vi "ActDriveStraight.vi"(9 "FirstTime":bool, 10 "MaxSpeed (ft/s)":dbl, 11 "Dist (ft)":dbl) -> (1 "XSpeedDemand":dbl, 3 "Done":bool)   [LabVIEW 2020]
doc: "Robot will drive forward straight a set distance utilizing position control \n\nInputs:\n-- MaxSpeed -- Double -- in ft/s, the MaxSpeed the robot can go -- \n-- Dist (ft) -- Double -- Distance in feet you want the robot to go -- \n-- FirstTime -- Boolean -- Input true the first time this function is called, sets the target position -- \n\nOutputs:\n-- Done -- Bool -- has the robot reached its target distance\n-- LeftSpeedDemand -- Double -- Speed Demand for left drive train inorder to reach target -- \n-- RightSpeedDemand -- Double -- Speed Demand for left drive train inorder to reach target --"
uses:
  <vilib>/Rock Robotics/WPI/ThirdParty/JAS_Junk/TrajLib/Trajectory_Library.lvlib
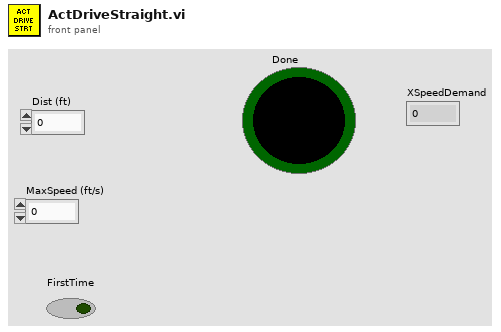
[diagram p1: front panel]
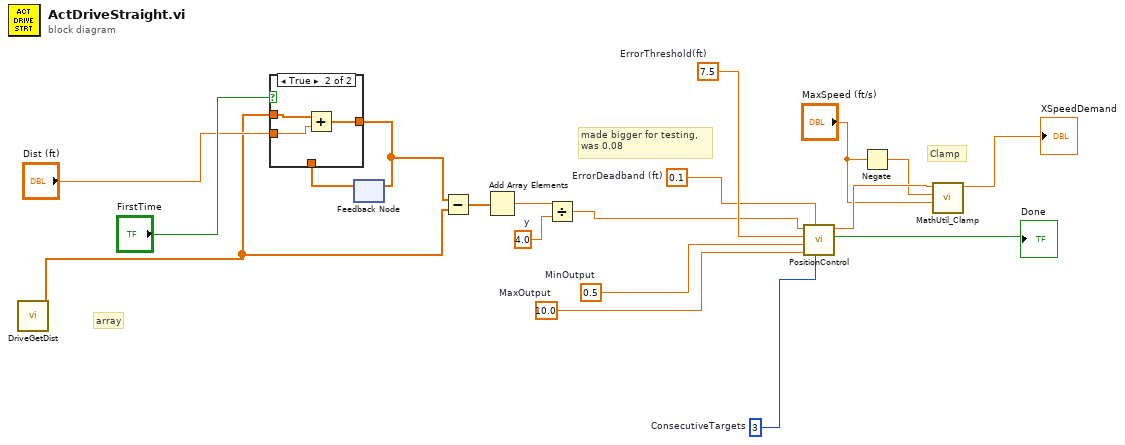
[diagram p0: block diagram]
diagram:
  w2 = 4.0  # y
  w10 = 10.0  # MaxOutput
  w11 = 0.5  # MinOutput
  w15 = 3  # ConsecutiveTargets
  w16 = 0.1  # ErrorDeadband (ft)
  w17 = 7.5  # ErrorThreshold(ft)
  # "made bigger for testing, \nwas 0.08"
  # "array"
  # "Clamp"
  n1 = call "DriveGetDist.vi"() -> ("ModuleTravelPosition"=w5:dbl[])  [unwired: 11 in]
  n2 = feedback #1() -> (w7:dbl[])  [unwired: 1 in]
  n3 = case shown="True" "FirstTime" {
    tunnel: "Dist (ft)" -> [_ w22]
    tunnel: w5 -> [_ w23]
    tunnel: [w20 w21] -> w6
    tunnel: w7 -> [w20 _]
    frame False {
    }
    frame True {
      n4 = Add(x=w23, y=w22) -> (x+y=w21:dbl[])
    }
  }
  n5 = feedback-in #1(w6) -> ()
  n6 = Subtract(x=w6, y=w5) -> (x-y=w4:dbl[])
  n7 = Add Array Elements(numeric array=w4) -> (sum=w3:dbl)
  n8 = Divide(x=w3, y=w2) -> (x/y=w1:dbl)
  n9 = call "PositionControl.vi"("ConsecutiveTargets"=w15, "ErrorDeadband"=w16, "MaxOutput"=w10, "MinOutput"=w11, "ErrorThreshold"=w17, "Error"=w1) -> ("OnTarget"=→"Done":bool, "OutputValue"=w14:dbl)  [unwired: 3 in, 1 out]
  n10 = Negate(x="MaxSpeed (ft/s)") -> (-x=w13:dbl)
  n11 = call <vilib>:"MathUtil_Clamp.vi"("High Limit"="MaxSpeed (ft/s)", "Low Limit"=w13, "Value"=w14) -> ("Result"=→"XSpeedDemand":dbl)  [unwired: 8 in]
